vi "VoltageUpdate.TestLauncher.vi"() -> ()   [LabVIEW 2016, in "VoltageUpdate.lvclass"]
uses:
  VoltageUpdate.lvclass
  <vilib>/JKI/JKI SMO/SMO/Typedefs/SMOState --Enum.ctl
  C:/Program Files (x86)/National Instruments/LabVIEW 2016/vi.lib/JKI/JKI SMO/SMO/SMO.lvclass
  C:/Program Files (x86)/National Instruments/LabVIEW 2016/user.lib/LevyLab/Levylab Instruments/SMOs/Instrument/Instrument.lvclass
  Program Files (x86)/National Instruments/LabVIEW 2016/templates/JKI/JKI SMO/Example Instrument UI/ExampleInstrumentUI.lvclass
  C:/Program Files (x86)/National Instruments/LabVIEW 2016/vi.lib/JKI/JKI SMO/SMO.UI/SMO.UI.lvclass
  <vilib>/JKI/JKI SMO/SMO/SMO.lvclass
  <vilib>/JKI/JKI SMO/SMO.UI/SMO.UI.lvclass
panel:
  out "UI SMO State":T1
  out "SMO State":T1
  out "error out":errorcluster
  in  "Stop":bool
  # "Example Instrument SMO Test Launcher"
  # "For instructions on how to use the JKI State Machine Objects, examples and video tutorials, visit:\nhttp://jki.net/state-machine-objects/\n\nJKI State Machine Objects™\nhttp://jki.net/state-machine-objects/\nCopyright (C) 2005-2015, JKI <info@jki.net>\nALL RIGHTS RESERVED"
  # "Starting Example Instrument..."
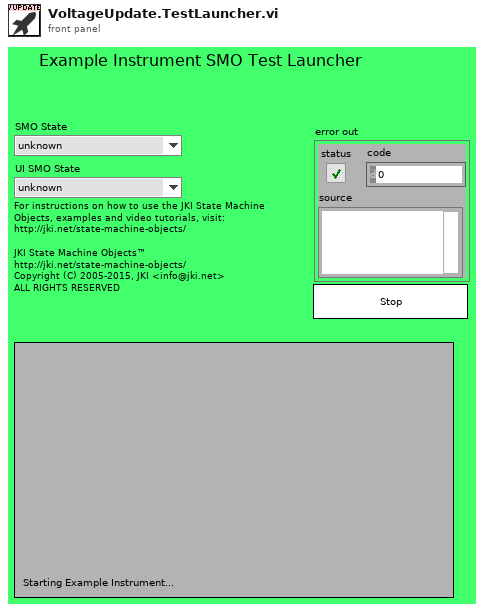
[diagram p1: front panel]
types:
  T1 = typedef "SMO.lvclass/SMOState --Enum.ctl" = enum16{"unknown", "Created", "Started", "Stopped"}
  T2 = typedef "SMO.lvclass/Public Events.ctl" = cluster{"Error":refnum<user-event>, "State":refnum<user-event>, "Reserve State":refnum<user-event>}
  T3 = cluster{"Event Registration Refnum":refnum<event-registration>, "Event Registration Refnum":refnum<event-registration>}
  T4 = enum32{"Invalid", "Standard", "Closed", "Hidden", "Minimized", "Maximized"}
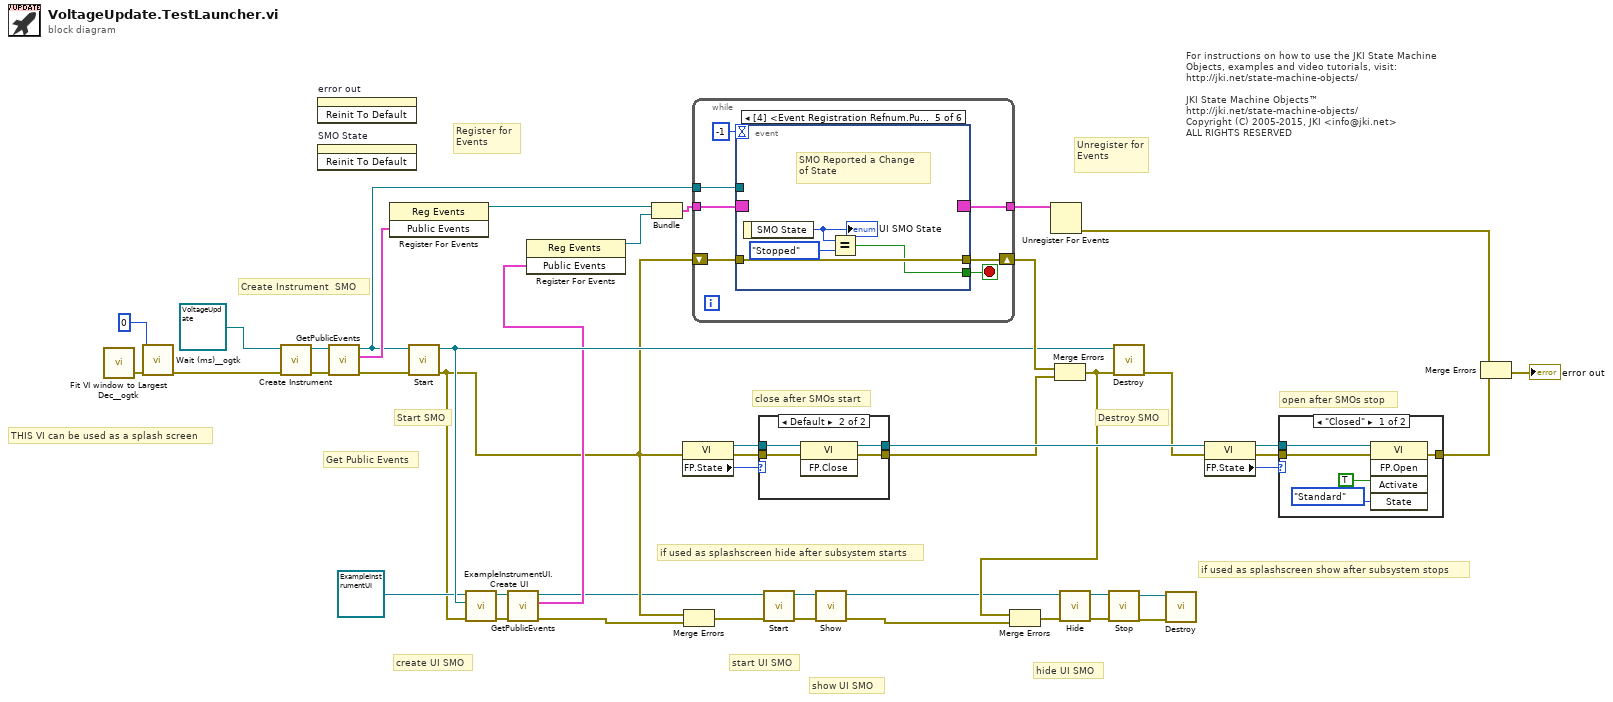
[diagram p0: block diagram]
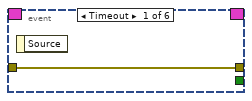
[diagram p4: hidden frame]
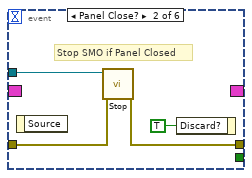
[diagram p5: hidden frame]
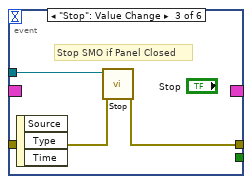
[diagram p6: hidden frame]
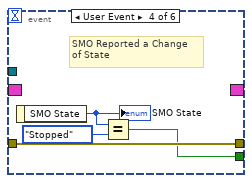
[diagram p7: hidden frame]
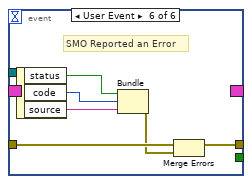
[diagram p8: hidden frame]
diagram:
  # "open after SMOs stop"
  # "close after SMOs start"
  # "hide UI SMO"
  # "show UI SMO"
  # "start UI SMO"
  # "create UI SMO"
  # "if used as splashscreen show after subsystem stops"
  # "if used as splashscreen hide after subsystem starts"
  # "THIS VI can be used as a splash screen"
  # "Get Public Events"
  # "Start SMO"
  # "Destroy SMO"
  # "Create Instrument  SMO"
  # "Unregister for Events"
  # "Register for Events"
  # "For instructions on how to use the JKI State Machine Objects, examples and video tutorials, visit:\nhttp://jki.net/state-machine-objects/\n\nJKI State Machine Objects™\nhttp://jki.net/state-machine-objects/\nCopyright (C) 2005-2015, JKI <info@jki.net>\nALL RIGHTS RESERVED"
  n1 = call <userlib>:"Fit VI window to Largest Dec__ogtk.vi"() -> ("error out"=w31:errorcluster)  [unwired: 6 in, 1 out]
  n2 = call <userlib>:"Wait (ms)__ogtk.vi"("error in (no error)"=w31, "milliseconds to wait"=u32 0) -> ("error out"=w2:errorcluster)  [unwired: 8 in, 1 out]
  n3 = call-dynamic "Create Instrument.vi"("error in (no error)"=w2, "Instrument in"=refnum<class "VoltageUpdate.lvclass"> refnum ("SMO.Template.lvclass")) -> ("error out"=w38:errorcluster, "Instrument out"=w39:refnum<class "VoltageUpdate.lvclass">)  [unwired: 8 in]
  n4 = invoke on="error out" class="Clust (strict)" method="Reinit To Default"() -> ()  [unwired: 3 in, 3 out]
  n5 = invoke on="SMO State" class="Enum (strict)" method="Reinit To Default"() -> ()  [unwired: 3 in, 3 out]
  n6 = call <vilib>:"GetPublicEvents.vi"("error in (no error)"=w38, "SMO"=w39) -> ("error out"=w37:errorcluster, "Public Events"=w41:T2, "SMO out"=w40:refnum<class "VoltageUpdate.lvclass">)  [unwired: 7 in]
  n7 = register-events(w41) -> (reference out=w30:refnum<event-registration>)  [unwired: 2 in, 1 out]
  n8 = call <vilib>:"Start.vi"("error in (no error)"=w37, "SMO"=w40) -> ("error out"=w22:errorcluster, "SMO out"=w28:refnum<class "VoltageUpdate.lvclass">)  [unwired: 8 in]
  n9 = call "ExampleInstrumentUI.Create UI.vi"("error in (no error)"=w22, "Instrument in"=w28, "Example Instrument UI in"=refnum<class "ExampleInstrumentUI.lvclass"> refnum ("Example Instrument UI.lvclass")) -> ("error out"=w25:errorcluster, "Example Instrument UI out"=w24:refnum<class "ExampleInstrumentUI.lvclass">)  [unwired: 7 in]
  n10 = call <vilib>:"GetPublicEvents.vi"("error in (no error)"=w25, "SMO"=w24) -> ("error out"=w16:errorcluster, "Public Events"=w23:T2, "SMO out"=w17:refnum<class "ExampleInstrumentUI.lvclass">)  [unwired: 7 in]
  n11 = register-events(w23) -> (reference out=w26:refnum<event-registration>)  [unwired: 2 in, 1 out]
  n12 = Bundle("Event Registration Refnum"=w30, "Event Registration Refnum"=w26) -> (w29:T3)  [unwired: 1 in]
  n13 = property class="VI"(error in=w22) -> (reference out=w7:refnum<vi>, error out=w8:errorcluster, "FP.State"=w6:T4)  [unwired: 1 in]
  n14 = Merge Errors(w22, w16) -> (w21:errorcluster)
  n15 = while {
    shift-right: [w51] -> w36
    shift-left: w22 -> [w50]
    tunnel: w29 -> [w49]
    tunnel: [w48] -> w44
    tunnel: w40 -> [w47]
    stop <- w52 stop-if-true
    n16 = event shown="[4] <Event Registration Refnum.Public Events.State>: User Event" {
      selector: w49 -> [_ _ _ _ _ _]
      dyn-events: [_ _ _ _ _ _] -> w48
      timeout: -1 -> [_ _ _ _ _ _]
      tunnel: [_ _ _ w61 w65 _] -> w52
      tunnel: w47 -> [_ w57 w60 _ _ _]
      tunnel: [w53 w56 w59 w64 w68 w72] -> w51
      tunnel: w50 -> [w53 w55 w58 w64 w68 w70]
      event Timeout {
        n17 = event-data() -> ()  [unwired: 1 in, 1 out]
      }
      event Panel Close? {
        # "Stop SMO if Panel Closed"
        n18 = event-data() -> ()  [unwired: 1 in, 1 out]
        n19 = call <vilib>:"Stop.vi"("error in (no error)"=w55, "SMO"=w57) -> ("error out"=w56:errorcluster)  [unwired: 8 in, 1 out]
        n20 = event-data("Discard?"=TRUE ("OK")) -> ()  [unwired: 1 in, 1 out]
      }
      event "Stop": Value Change {
        # "Stop SMO if Panel Closed"
        n21 = event-data() -> ()  [unwired: 1 in, 3 out]
        n22 = call <vilib>:"Stop.vi"("error in (no error)"=w58, "SMO"=w60) -> ("error out"=w59:errorcluster)  [unwired: 8 in, 1 out]
      }
      event User Event {
        # "SMO Reported a Change\nof State"
        n23 = event-data() -> ("SMO State"=w63:T1)  [unwired: 1 in]
        "SMO State" <- w63
        n24 = Equal?(x=w63, y=SMOState_--Enum."Stopped") -> (x = y?=w61:bool)
      }
      event User Event {
        # "SMO Reported a Change\nof State"
        n25 = event-data() -> ("SMO State"=w67:T1)  [unwired: 1 in]
        "UI SMO State" <- w67
        n26 = Equal?(x=w67, y=SMOState_--Enum."Stopped") -> (x = y?=w65:bool)
      }
      event User Event {
        # "SMO Reported an Error"
        n27 = event-data() -> ("status"=w71:bool, "code"=w74:i32, "source"=w73:string)  [unwired: 1 in]
        n28 = Bundle("status"=w71, "code"=w74, "source"=w73) -> (w69:errorcluster)  [unwired: 1 in]
        n29 = Merge Errors(w70, w69) -> (w72:errorcluster)
      }
    }
  }
  n30 = case shown="Default" w6 {
    tunnel: [w76 w80] -> w32
    tunnel: w8 -> [w76 w79]
    tunnel: w7 -> [w75 w78]
    tunnel: [w75 w77] -> w35
    frame "Invalid", "Closed" {
    }
    frame Default {
      n31 = invoke class="VI" method="FP.Close"(reference=w78, error in=w79) -> (reference out=w77:refnum<vi>, error out=w80:errorcluster)  [unwired: 1 in, 1 out]
    }
  }
  n32 = call <vilib>:"Start.vi"("error in (no error)"=w21, "SMO"=w17) -> ("error out"=w15:errorcluster, "SMO out"=w14:refnum<class "ExampleInstrumentUI.lvclass">)  [unwired: 8 in]
  n33 = call <vilib>:"Show.vi"("error in (no error)"=w15, "SMO.UI"=w14) -> ("error out"=w13:errorcluster, "SMO.UI out"=w9:refnum<class "ExampleInstrumentUI.lvclass">)  [unwired: 8 in]
  n34 = Unregister For Events(event registration refnum=w44) -> (error out=w43:errorcluster)  [unwired: 1 in]
  n35 = Merge Errors(w36, w32) -> (w18:errorcluster)
  n36 = Merge Errors(w18, w13) -> (w10:errorcluster)
  n37 = call <vilib>:"Hide.vi"("error in (no error)"=w10, "SMO.UI"=w9) -> ("error out"=w12:errorcluster, "SMO.UI out"=w11:refnum<class "ExampleInstrumentUI.lvclass">)  [unwired: 8 in]
  n38 = call <vilib>:"Stop.vi"("error in (no error)"=w12, "SMO"=w11) -> ("error out"=w20:errorcluster, "SMO out"=w19:refnum<class "ExampleInstrumentUI.lvclass">)  [unwired: 8 in]
  n39 = call <vilib>:"Destroy.vi"("error in (no error)"=w18, "SMO"=w28) -> ("error out"=w34:errorcluster)  [unwired: 9 in]
  n40 = call <vilib>:"Destroy.vi"("error in (no error)"=w20, "SMO"=w19) -> ()  [unwired: 9 in, 1 out]
  n41 = property class="VI"(reference=w35, error in=w34) -> (reference out=w4:refnum<vi>, error out=w5:errorcluster, "FP.State"=w3:T4)
  n42 = case shown="\"Closed\"" w3 {
    tunnel: [w83 w86] -> w33
    tunnel: w5 -> [w82 w86]
    tunnel: w4 -> [w81 _]
    frame "Closed" {
      n43 = invoke class="VI" method="FP.Open"(reference=w81, error in=w82, "Activate"=TRUE, "State"=T4."Standard") -> (error out=w83:errorcluster)  [unwired: 1 in, 4 out]
    }
    frame Default {
    }
  }
  n44 = Merge Errors(w43, w33) -> (→"error out":errorcluster)
